vi "FormatPoint.vi"(1 "point":T1) -> (0 "value":string)   [LabVIEW 2014, in "PythonConfiguration.lvclass"]
uses:
  PythonConfiguration.lvclass
  <vilib>/Utility/miscctls.llb/LVPointTypeDef.ctl
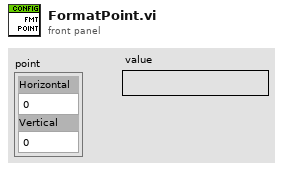
[diagram p1: front panel]
types:
  T1 = typedef "LVPointTypeDef.ctl" = cluster{"Horizontal":i16, "Vertical":i16}
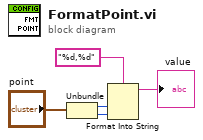
[diagram p0: block diagram]
diagram:
  n1 = Unbundle("point") -> ("Horizontal"=w4:i16, "Vertical"=w3:i16)
  n2 = Format Into String(format string="%d,%d", w4, w3) -> (resulting string=→"value":string)  [unwired: 2 in, 1 out]
